vi "SetConfig.vi"(0 "class data in":refnum<class "AbruptChange.lvclass">, 5 "SettinganalogComp":T1, 7 "default value":dbl, 9 "size (10)":u32, 11 "error in (no error)":errorcluster) -> (4 "class data out":refnum<class "AbruptChange.lvclass">, 15 "error out":errorcluster)   [LabVIEW 2019, in "AbruptChange.lvclass"]
uses:
  AbruptChange.lvclass
  TypeDef/ConfigAnalogComp.ctl
  AbruptChange.lvclass/AbruptChange.ctl
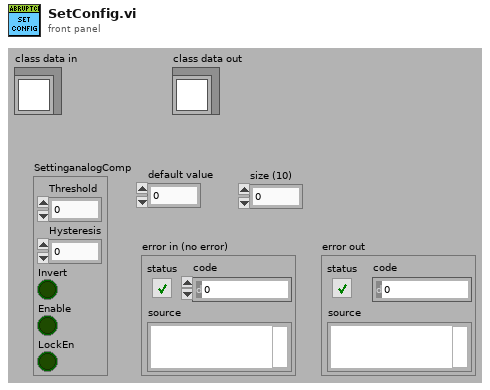
[diagram p1: front panel]
types:
  T1 = typedef "ConfigAnalogComp.ctl" = cluster{"Threshold":dbl, "Hysteresis":dbl, "Invert":bool, "Enable":bool, "LockEn":bool}
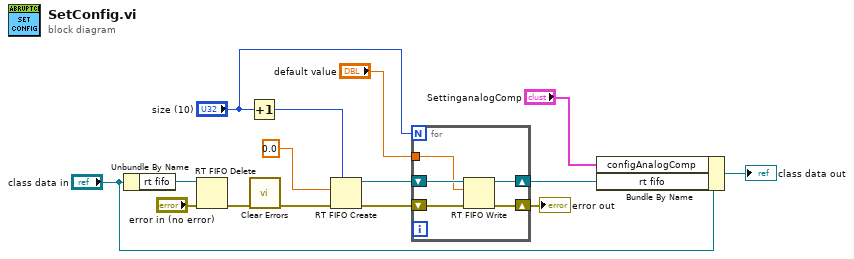
[diagram p0: block diagram]
diagram:
  n1 = Unbundle By Name("class data in") -> ("rt fifo"=w4:refnum<k33>)
  n2 = RT FIFO Delete(0:w4, 3:"error in (no error)") -> (11:w12:errorcluster)  [unwired: 1 in]
  n3 = Increment(x="size (10)") -> (x+1=w10:u32)
  n4 = call <vilib>:"Clear Errors.vi"("error in (no error)"=w12) -> ("error out"=w11:errorcluster)  [unwired: 5 in, 1 out]
  n5 = RT FIFO Create(1:0.0, 3:w11, 4:w10) -> (8:w9:refnum<k33>, 11:w8:errorcluster)  [unwired: 5 in, 1 out]
  n6 = for {
    N: "size (10)" -> [_]
    shift-right: [w19] -> w3
    shift-left: w9 -> [w20]
    shift-right: [w17] -> w1
    shift-left: w8 -> [w18]
    tunnel: "default value" -> [w16]
    n7 = RT FIFO Write(0:w20, 1:w16, 3:w18) -> (8:w19:refnum<k33>, 11:w17:errorcluster)  [unwired: 2 in, 2 out]
  }
  "error out" <- w1
  n8 = Bundle By Name(cluster="class data in", "configAnalogComp"="SettinganalogComp", "rt fifo"=w3) -> (→"class data out":refnum<class "AbruptChange.lvclass">)
